vi "Is status ongoing.vi"   [LabVIEW 2020, in "TALOS.lvlib" / "Tamer.lvlib" / "Tamer.lvclass"]
uses:
  Tamer.lvclass
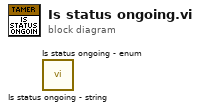
[diagram p0: block diagram]
diagram:
  n1 = call "Is status ongoing - string.vi"() -> ()  [unwired: 1 in, 1 out]
  n2 = call "Is status ongoing - enum.vi"() -> ()  [unwired: 1 in, 1 out]
